vi "Configure Bit Error Rate Polarity.vi"(8 "error in (no error)":errorcluster, 9 "Input Polarity (0: Positive)":i32(ring) items=["Positive", "Negative"], 10 "Signal Supply (0: Gate)":i32(ring) items=["Gate", "Clock", "Data"], 11 "VISA resource name":refnum<visa-resource-name>) -> (0 "error out":errorcluster, 3 "VISA resource name out":refnum<visa-resource-name>)   [LabVIEW 2018, in "Agilent PSG MXG Series.lvlib"]
doc: "Configures the input polarity of the clock, data and gate signal supplied.\n\n<b>Note:</b>\nIt is applicable for N5172B/82B with <b>Option UN7</b> only."
uses:
  Agilent PSG MXG Series.lvlib
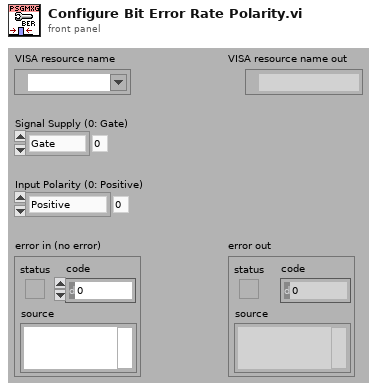
[diagram p1: front panel]
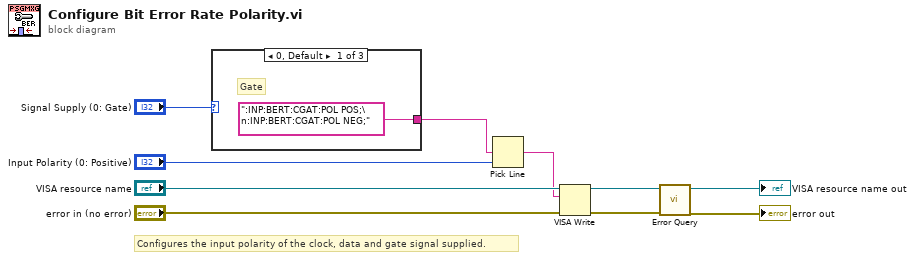
[diagram p0: block diagram]
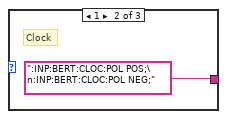
[diagram p2: hidden frame]
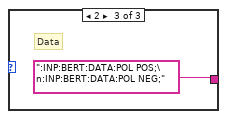
[diagram p3: hidden frame]
diagram:
  # "Configures the input polarity of the clock, data and gate signal supplied."
  n1 = case shown="0, Default" "Signal Supply (0: Gate)" {
    tunnel: [":INP:BERT:CGAT:POL POS;\n:INP:BERT:CGAT:POL NEG;" ":INP:BERT:CLOC:POL POS;\n:INP:BERT:CLOC:POL NEG;" ":INP:BERT:DATA:POL POS;\n:INP:BERT:DATA:POL NEG;"] -> w1
    frame 0, Default {
      # "Gate"
    }
    frame 1 {
      # "Clock"
    }
    frame 2 {
      # "Data"
    }
  }
  n2 = Pick Line(multi-line string=w1, line index="Input Polarity (0: Positive)") -> (output string=w3:string)  [unwired: 1 in]
  n3 = VISA Write(VISA resource name="VISA resource name", write buffer=w3, error in (no error)="error in (no error)") -> (VISA resource name out=w8:refnum<visa-resource-name>, error out=w7:errorcluster)  [unwired: 1 out]
  n4 = call "Error Query.vi"("error in (no error)"=w7, "VISA resource name"=w8) -> ("error out"=→"error out":errorcluster, "VISA resource name out"=→"VISA resource name out":refnum<visa-resource-name>)  [unwired: 6 in, 2 out]
